vi "Set Pending Operation.vi"(8 "error in":errorcluster, 11 "Remote Operation Abstract":refnum<class "Remote Operation Abstract.lvclass">) -> (0 "error out":errorcluster, 3 "dup Remote Operation Abstract":refnum<class "Remote Operation Abstract.lvclass">)   [LabVIEW 2018, in "Remote Operation Abstract.lvlib" / "Remote Operation Abstract.lvclass"]
uses:
  Remote Operation Abstract.lvclass
  Remote Operation Abstract.lvclass/Remote Operation Abstract.ctl
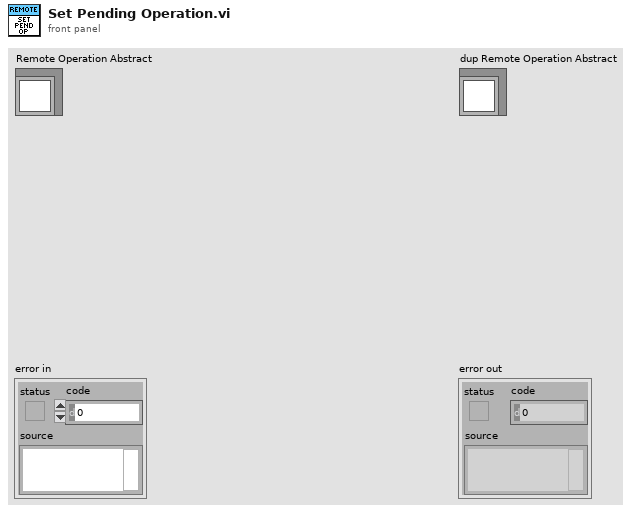
[diagram p1: front panel]
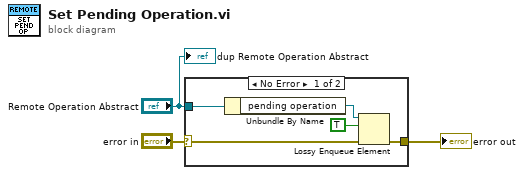
[diagram p0: block diagram]
diagram:
  n1 = case shown="No Error" "error in" {
    selector: "error in" -> [w7 w9]
    tunnel: [w6 w9] -> w2
    tunnel: "Remote Operation Abstract" -> [w8 _]
    frame No Error {
      n2 = Unbundle By Name(w8) -> ("pending operation"=w5:refnum<queue>)
      n3 = Lossy Enqueue Element(queue=w5, element=TRUE, error in (no error)=w7) -> (error out=w6:errorcluster)  [unwired: 3 out]
    }
    frame Error {
    }
  }
  "error out" <- w2
  "dup Remote Operation Abstract" <- "Remote Operation Abstract"
